vi "Get Saving Data Path.vi"(10 "L_Or_R":bool, 11 "Measure_ID":i32) -> ()   [LabVIEW 2015, in "Utility VIs.lvlib"]
uses:
  Utility VIs.lvlib
panel:
  out "Get Saving Data":T1
  in  "Ordinal Right":i32
  in  "Ordinal Left":i32
  in  "Measure_No":i32
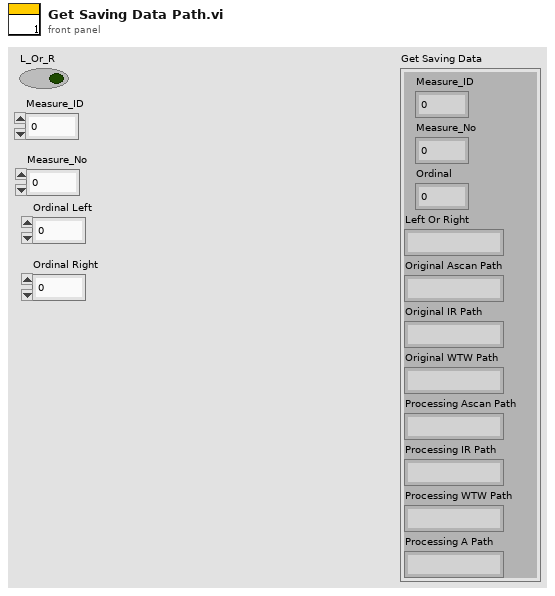
[diagram p1: front panel]
types:
  T1 = cluster{"Measure_ID":i32, "Measure_No":i32, "Ordinal":i32, "Left Or Right":string, "Original Ascan Path":string, "Original IR Path":string, "Original WTW Path":string, "Processing Ascan Path":string, "Processing IR Path":string, "Processing WTW Path":string, "Processing A Path":string}
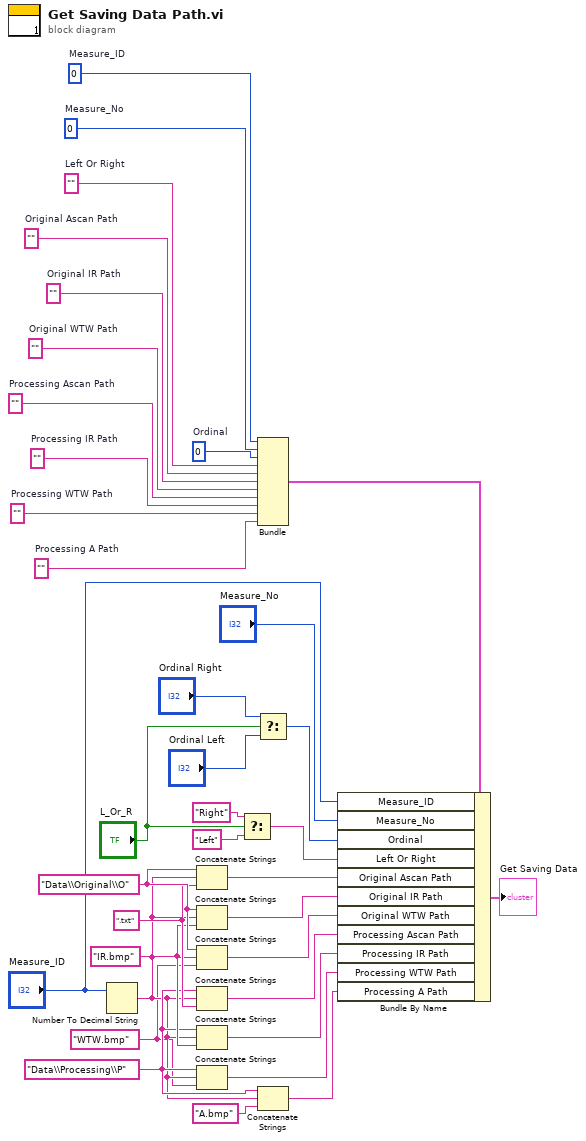
[diagram p0: block diagram]
diagram:
  w9 = 0  # Measure_ID
  w10 = 0  # Measure_No
  w11 = 0  # Ordinal
  w12 = ""  # Left Or Right
  w21 = ""  # Processing A Path
  w22 = ""  # Processing WTW Path
  w23 = ""  # Processing IR Path
  w24 = ""  # Processing Ascan Path
  w25 = ""  # Original WTW Path
  w26 = ""  # Original IR Path
  w27 = ""  # Original Ascan Path
  w31 = "Data\\Processing\\P"
  w29 = "WTW.bmp" ("字符串")
  w32 = "IR.bmp" ("字符串")
  w33 = ".txt" ("字符串")
  w36 = "Data\\Original\\O"
  n1 = Number To Decimal String(number="Measure_ID") -> (decimal integer string=w30:string)  [unwired: 1 in]
  n2 = Concatenate Strings(w36, w30, w33) -> (w19:string)
  n3 = Concatenate Strings(w36, w30, w32) -> (w18:string)
  n4 = Concatenate Strings(w36, w30, w29) -> (w17:string)
  n5 = Concatenate Strings(w31, w30, w33) -> (w16:string)
  n6 = Concatenate Strings(w31, w30, w32) -> (w15:string)
  n7 = Concatenate Strings(w31, w30, w29) -> (w14:string)
  n8 = Select(t="Right" ("字符串"), s="L_Or_R", f="Left" ("字符串")) -> (s? t:f=w8:string)
  n9 = Bundle("Measure_ID"=w9, "Measure_No"=w10, "Ordinal"=w11, "Left Or Right"=w12, "Original Ascan Path"=w27, "Original IR Path"=w26, "Original WTW Path"=w25, "Processing Ascan Path"=w24, "Processing IR Path"=w23, "Processing WTW Path"=w22, "Processing A Path"=w21) -> (w20:T1)  [unwired: 1 in]
  n10 = Select(t="Ordinal Right", s="L_Or_R", f="Ordinal Left") -> (s? t:f=w2:i32)
  n11 = Concatenate Strings(w31, w30, "A.bmp" ("字符串")) -> (w13:string)
  n12 = Bundle By Name(cluster=w20, "Measure_ID"="Measure_ID", "Measure_No"="Measure_No", "Ordinal"=w2, "Left Or Right"=w8, "Original Ascan Path"=w19, "Original IR Path"=w18, "Original WTW Path"=w17, "Processing Ascan Path"=w16, "Processing IR Path"=w15, "Processing WTW Path"=w14, "Processing A Path"=w13) -> (→"Get Saving Data":T1)
